vi "Menu-Start Log EOC.vi"(11 "Menu in":refnum<k9>) -> ()   [LabVIEW 2016, in "CML UI.lvlib"]
uses:
  CML UI.lvlib
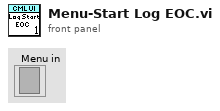
[diagram p1: front panel]
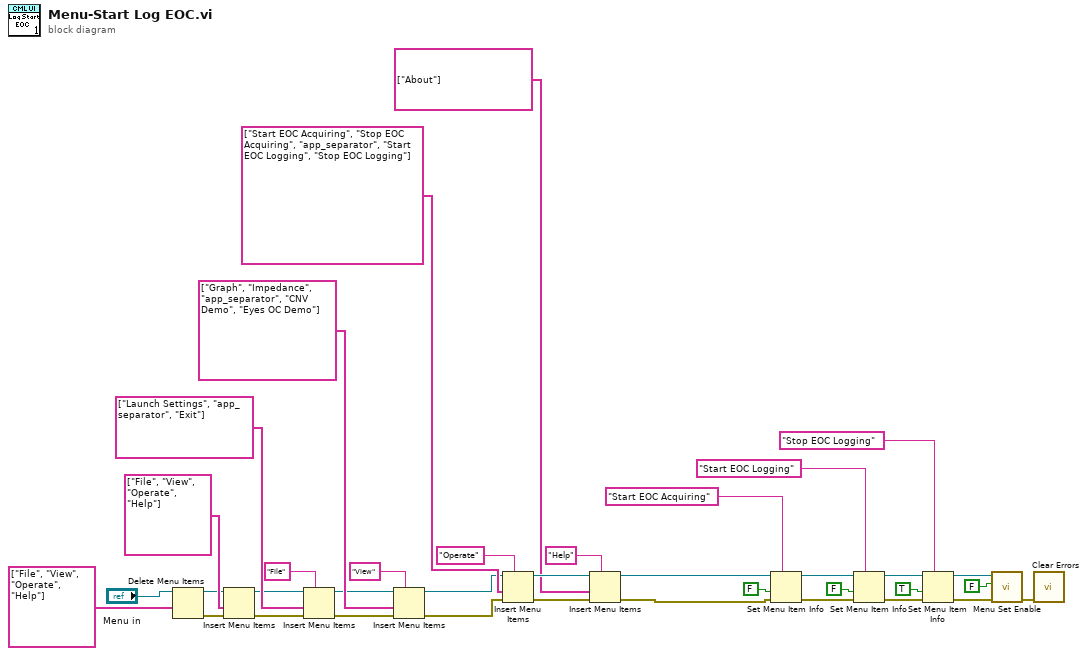
[diagram p0: block diagram]
diagram:
  n1 = Delete Menu Items(7:string[] ["File", "View", "Operate", "Help"] ("L10n_item tags 1"), 9:"Menu in") -> (0:w14:errorcluster, 3:w15:refnum<k9>)  [unwired: 2 in]
  n2 = Insert Menu Items(6:w14, 7:string[] ["File", "View", "Operate", "Help"] ("L10n_item tags 1"), 9:w15) -> (0:w26:errorcluster, 3:w24:refnum<k9>)  [unwired: 3 in, 1 out]
  n3 = Insert Menu Items(5:"File" ("L10n_menu tag"), 6:w26, 7:string[] ["Launch Settings", "app_separator", "Exit"] ("L10n_item tags 2"), 9:w24) -> (0:w31:errorcluster, 3:w30:refnum<k9>)  [unwired: 2 in, 1 out]
  n4 = Insert Menu Items(5:"View" ("L10n_menu tag"), 6:w31, 7:string[] ["Graph", "Impedance", "app_separator", "CNV Demo", "Eyes OC Demo"] ("L10n_item tags 2"), 9:w30) -> (0:w35:errorcluster, 3:w34:refnum<k9>)  [unwired: 2 in, 1 out]
  n5 = Insert Menu Items(5:"Operate" ("L10n_menu tag"), 6:w35, 7:string[] ["Start EOC Acquiring", "Stop EOC Acquiring", "app_separator", "Start EOC Logging", "Stop EOC Logging"] ("L10n_item tags 2"), 9:w34) -> (0:w21:errorcluster, 3:w22:refnum<k9>)  [unwired: 2 in, 1 out]
  n6 = Insert Menu Items(5:"Help" ("L10n_menu tag"), 6:w21, 7:string[] ["About"] ("L10n_item tags 2"), 9:w22) -> (0:w18:errorcluster, 3:w19:refnum<k9>)  [unwired: 2 in, 1 out]
  n7 = Set Menu Item Info(7:"Start EOC Acquiring" ("item tag"), 8:w18, 9:FALSE ("enabled"), 11:w19) -> (0:w8:errorcluster, 3:w9:refnum<k9>)  [unwired: 3 in]
  n8 = Set Menu Item Info(7:"Start EOC Logging" ("item tag"), 8:w8, 9:FALSE ("enabled"), 11:w9) -> (0:w6:errorcluster, 3:w7:refnum<k9>)  [unwired: 3 in]
  n9 = Set Menu Item Info(7:"Stop EOC Logging" ("item tag"), 8:w6, 9:TRUE ("enabled"), 11:w7) -> (0:w4:errorcluster, 3:w3:refnum<k9>)  [unwired: 3 in]
  n10 = call "Menu Set Enable.vi"("error in (no error)"=w4, "enabled ?"=FALSE, "Menu in"=w3) -> ("error out"=w2:errorcluster)  [unwired: 7 in, 1 out]
  n11 = call <vilib>:"Clear Errors.vi"("error in (no error)"=w2) -> ()  [unwired: 5 in, 2 out]
